vi "Get TempSP.vi"(8 "error in (no error)":errorcluster, 11 "Modbus Master in":refnum<class "Modbus Master.lvclass">) -> (0 "error out":errorcluster, 2 "SetPoint (C)":dbl, 3 "Modbus Master out":refnum<class "Modbus Master.lvclass">)   [LabVIEW 2023, in "PIDModbus.lvlib"]
uses:
  PIDModbus.lvlib
  <vilib>/NI/Modbus Library/API/Master/Modbus Master.lvclass
  Controls/Register Enum.ctl
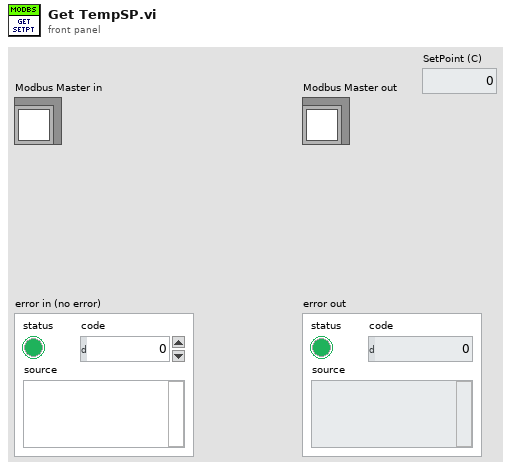
[diagram p1: front panel]
types:
  T1 = typedef "PIDModbus.lvlib/Register Enum.ctl" = u16
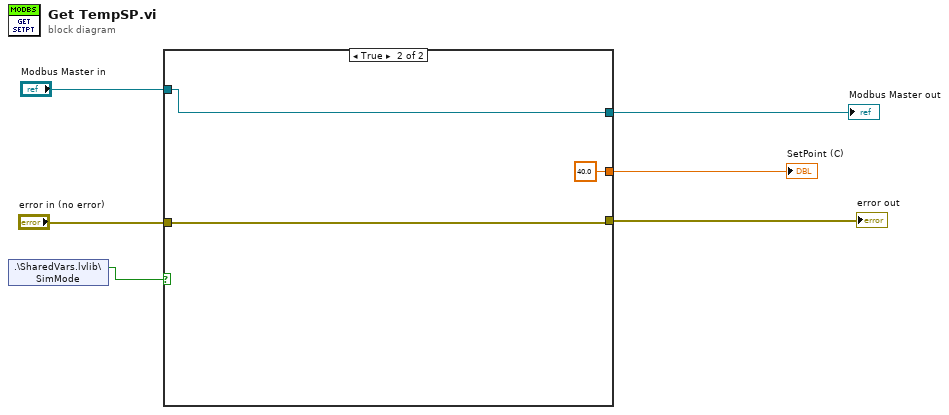
[diagram p0: block diagram]
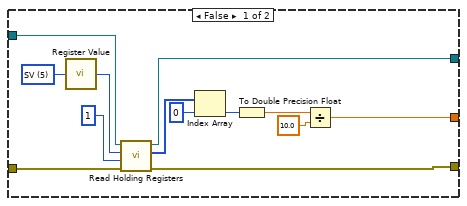
[diagram p2: hidden frame]
diagram:
  n1 = shared-variable ".\\SharedVars.lvlib\\SimMode"() -> (w1:bool)  [unwired: 1 in, 1 out]
  n2 = case shown="True" w1 {
    tunnel: [w19 w20] -> w6
    tunnel: [w18 w22] -> w5
    tunnel: "error in (no error)" -> [w15 w20]
    tunnel: "Modbus Master in" -> [w14 w22]
    tunnel: [w7 40.0] -> w2
    frame False {
      w13 = T1 5 items=["PV"=0, "SV"=5, "P1"=24, "I1"=25, "D1"=26] ("Register")
      n3 = call "Register Value.vi"("Register"=w13) -> ("RegAddr (Hex)"=w12:u16)
      n4 = call-dynamic "Read Holding Registers.vi"("error in"=w15, "number of inputs"=u16 1, "starting address"=w12, "Modbus master in"=w14) -> ("error out"=w19:errorcluster, "register values"=w17:u16[], "Modbus master out"=w18:refnum<class "Modbus Master.lvclass">)  [unwired: 5 in]
      n5 = Index Array(array=w17, index=0) -> (element=w10:u16)
      n6 = To Double Precision Float(number=w10) -> (double precision float=w8:dbl)
      n7 = Divide(x=w8, y=10.0) -> (x/y=w7:dbl)
    }
    frame True {
    }
  }
  "error out" <- w6
  "Modbus Master out" <- w5
  "SetPoint (C)" <- w2
